vi "Test_Reactor_Coolant_Pump_Motor_Speed_Loop.vi.vi"() -> ()   [LabVIEW 2022 SP3]
uses:
  SI_modules/SI600/SI600.lvclass
panel:
  out "RCP Spped Loop":cluster{"Time":timestamp[], dbl[]}(graph)
  out "Inputs":cluster{"Time":timestamp[], dbl[]}[](graph)
  out "Outputs":cluster{"Time":timestamp[], dbl[]}[](graph)
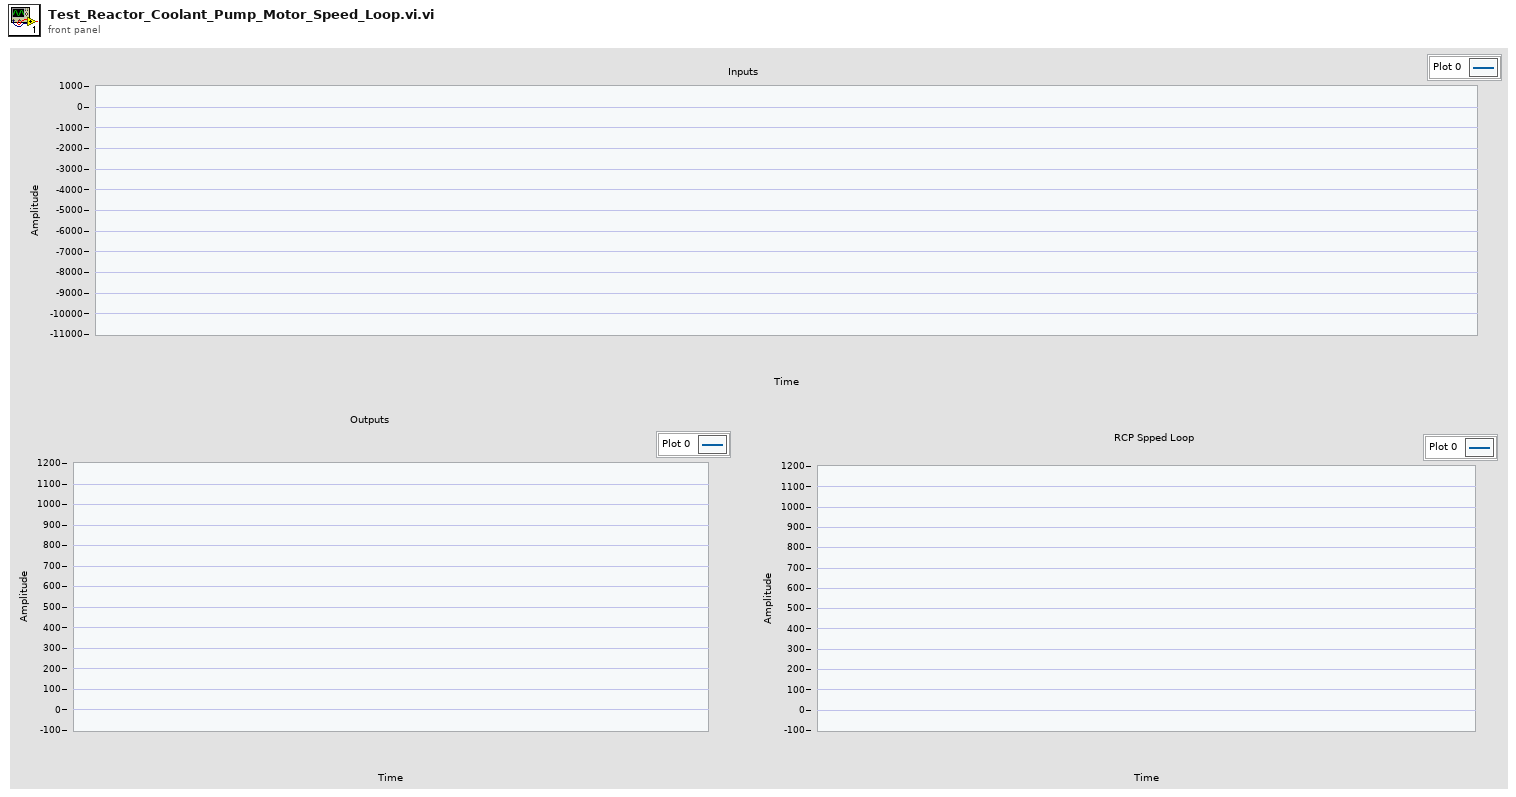
[diagram p1: front panel]
types:
  T1 = cluster{"[0]":cluster{"Time":timestamp[], "KKS":string, "Meas":dbl[]}, "[1]":cluster{"Time":timestamp[], "KKS":string, "Meas":dbl[]}, "[2]":cluster{"Time":timestamp[], "KKS":string, "Meas":dbl[]}, "[3]":cluster{"Time":timestamp[], "KKS":string, "Meas":dbl[]}, "[4]":cluster{"Time":timestamp[], "KKS":string, "Meas":dbl[]}, "[5]":cluster{"Time":timestamp[], "KKS":string, "Meas":dbl[]}, "[6]":cluster{"Time":timestamp[], "KKS":string, "Meas":dbl[]}, "[7]":cluster{"Time":timestamp[], "KKS":string, "Meas":dbl[]}, "[8]":cluster{"Time":timestamp[], "KKS":string, "Meas":dbl[]}}
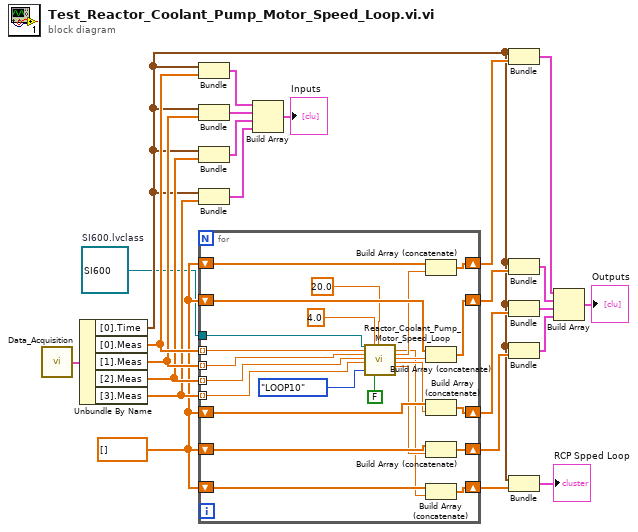
[diagram p0: block diagram]
diagram:
  w1 = refnum<class "SI600.lvclass"> refnum  # SI600.lvclass
  w5 = dbl[] []
  n1 = call "Data_Acquisition.vi"() -> ("Meas"=w24:T1)  [unwired: 15 in]
  n2 = Unbundle By Name(w24) -> ("[0].Time"=w3:timestamp[], "[0].Meas"=w14:dbl[], "[1].Meas"=w13:dbl[], "[2].Meas"=w12:dbl[], "[3].Meas"=w11:dbl[])
  n3 = Bundle("Time"=w3, "Meas"=w14) -> (w10:cluster{"Time":timestamp[], "Meas":dbl[]})  [unwired: 1 in]
  n4 = Bundle("Time"=w3, "Meas"=w13) -> (w9:cluster{"Time":timestamp[], "Meas":dbl[]})  [unwired: 1 in]
  n5 = Bundle("Time"=w3, "Meas"=w12) -> (w8:cluster{"Time":timestamp[], "Meas":dbl[]})  [unwired: 1 in]
  n6 = Bundle("Time"=w3, "Meas"=w11) -> (w7:cluster{"Time":timestamp[], "Meas":dbl[]})  [unwired: 1 in]
  n7 = for {
    tunnel: w1 -> [w39]
    tunnel: w14 -> [w38] mode=indexing
    tunnel: w13 -> [w37] mode=indexing
    tunnel: w12 -> [w36] mode=indexing
    tunnel: w11 -> [w35] mode=indexing
    shift-right: [w48] -> w23
    shift-left: w5 -> [w44]
    shift-right: [w47] -> w22
    shift-left: w5 -> [w43]
    shift-right: [w46] -> w21
    shift-left: w5 -> [w42]
    shift-right: [w45] -> w20
    shift-left: w5 -> [w41]
    shift-right: [w28] -> w4
    shift-left: w5 -> [w40]
    n8 = call "Reactor_Coolant_Pump_Motor_Speed_Loop.vi"("SI600.lvclass in"=w39, "3 JEB CS951 XQ01"=w38, "3 JEB CS952 XQ01"=w37, "3 JEB CS953 XQ01"=w36, "3 JEB CS954 XQ01"=w35, "Loop"=enum16{"LOOP10", "LOOP20", "LOOP30", "LOOP40"}."LOOP10", "In1"=4.0, "Limitation"=FALSE, "In2"=20.0) -> ("RCP speed Loop Output"=w29:dbl, "3 JEB CS951"=w33:dbl, "3 JEB CS952"=w32:dbl, "3 JEB CS953"=w31:dbl, "3 JEB CS954"=w30:dbl)  [unwired: 12 in, 2 out]
    n9 = Build Array (concatenate)(w44, w33) -> (w48:dbl[])
    n10 = Build Array (concatenate)(w43, w32) -> (w47:dbl[])
    n11 = Build Array (concatenate)(w42, w31) -> (w46:dbl[])
    n12 = Build Array (concatenate)(w41, w30) -> (w45:dbl[])
    n13 = Build Array (concatenate)(w40, w29) -> (w28:dbl[])
  }
  n14 = Build Array(w10, w9, w8, w7) -> (→"Inputs":cluster{"Time":timestamp[], "Meas":dbl[]}[])
  n15 = Bundle("Time"=w3, w23) -> (w19:cluster{"Time":timestamp[], dbl[]})  [unwired: 1 in]
  n16 = Bundle("Time"=w3, w22) -> (w18:cluster{"Time":timestamp[], dbl[]})  [unwired: 1 in]
  n17 = Bundle("Time"=w3, w21) -> (w17:cluster{"Time":timestamp[], dbl[]})  [unwired: 1 in]
  n18 = Bundle("Time"=w3, w20) -> (w16:cluster{"Time":timestamp[], dbl[]})  [unwired: 1 in]
  n19 = Bundle("Time"=w3, w4) -> (→"RCP Spped Loop":cluster{"Time":timestamp[], dbl[]})  [unwired: 1 in]
  n20 = Build Array(w19, w18, w17, w16) -> (→"Outputs":cluster{"Time":timestamp[], dbl[]}[])
